vi "Coherent command pst-processing L1.vi"(6 "Data Type":T1, 7 "Coherent laser commands L1":T2(ring)=enum."Set Command", 8 "error in (no error)":errorcluster, 9 "Command Validated":bool, 10 "Response String":string, 11 "Command String":string) -> (0 "error out":errorcluster, 1 "Response String":string, 2 "Data Type":T1, 3 "trimmed string":string)   [LabVIEW 2020]
uses:
  Type defs/data type.ctl
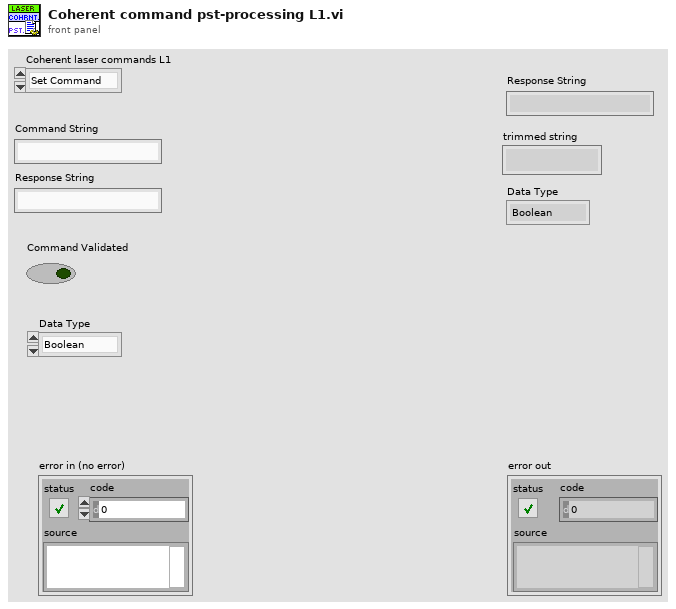
[diagram p1: front panel]
types:
  T1 = typedef "data type.ctl" = enum16{"Boolean", "Flag", "Numeric", "String", "Array"}
  T2 = enum16{"Initialise", "Get Command", "Set Command", "Close"}
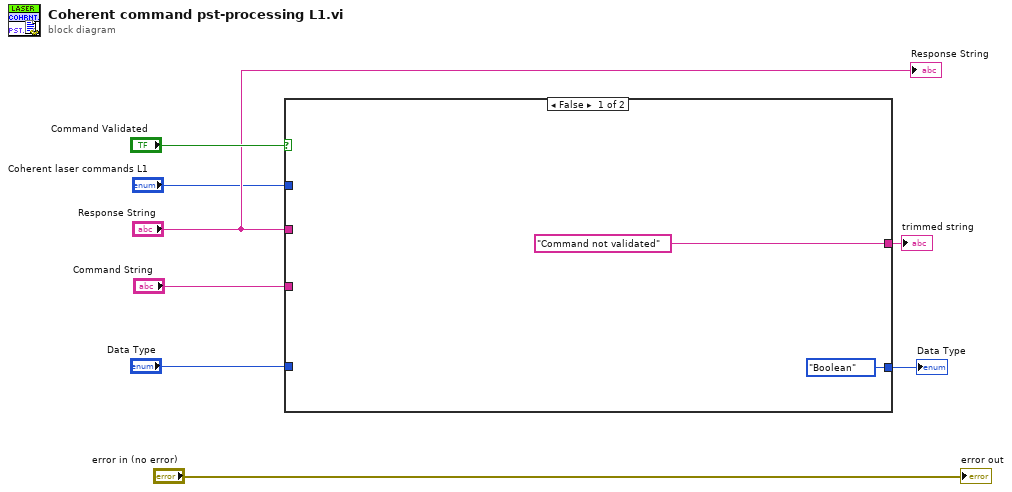
[diagram p0: block diagram]
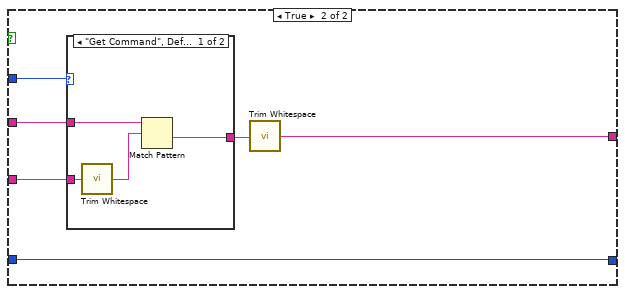
[diagram p2: hidden frame]
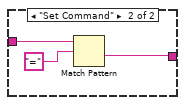
[diagram p3: hidden frame]
diagram:
  n1 = case shown="False" "Command Validated" {
    tunnel: "Response String" -> [_ w15]
    tunnel: "Data Type" -> [_ w12]
    tunnel: "Coherent laser commands L1" -> [_ w16]
    tunnel: "Command String" -> [_ w14]
    tunnel: [data_type."Boolean" ("Data Type") w12] -> w3
    tunnel: ["Command not validated" ("String") w11] -> w1
    frame False {
    }
    frame True {
      n2 = case shown="\"Get Command\", Default" w16 {
        tunnel: w15 -> [w20 w23]
        tunnel: w14 -> [w18 _]
        tunnel: [w19 w21] -> w13
        frame "Get Command", Default {
          n3 = call <vilib>:"Trim Whitespace.vi"("string"=w18) -> ("trimmed string"=w17:string)  [unwired: 1 in]
          n4 = Match Pattern(string=w20, regular expression=w17) -> (after substring=w19:string)  [unwired: 1 in, 3 out]
        }
        frame "Set Command" {
          n5 = Match Pattern(string=w23, regular expression="=") -> (after substring=w21:string)  [unwired: 1 in, 3 out]
        }
      }
      n6 = call <vilib>:"Trim Whitespace.vi"("string"=w13) -> ("trimmed string"=w11:string)  [unwired: 1 in]
    }
  }
  "Data Type" <- w3
  "trimmed string" <- w1
  "Response String" <- "Response String"
  "error out" <- "error in (no error)"
